vi "Gantry_GUI_Events.vi"(0 "COMPORT":refnum<visa-resource-name>="COM5", 5 "error in (no error)":errorcluster, 7 "Antenna Select":u16(ring)=1 items=["HOME", "TX1", "TX2", "TX3", "TX4", "TX5", "TX6", "TX7", "TX8", "TX9", "TX10", "TX11", "TX12", "RX8", "RX7", "RX6", "RX5", "RX4", "RX3", "RX2", "RX1"], 8 "EnableDriver(t)":bool=TRUE, 9 "z ref":dbl=21.0 format="%#_6f", 10 "Operation":u16(ring) items=["W/R", "RD ONLY", "WR ONLY"], 11 "Set-Z(Inches)":dbl=21.0 format="%#_6f") -> (14 "GantryGuiRefOut":refnum<vi>, 19 "error out":errorcluster)   [LabVIEW 2018]
uses:
  <vilib>/Utility/file.llb/Read Delimited Spreadsheet (DBL).vi
panel:
  in  "Exe_write":bool=TRUE
  in  "Exit":bool=TRUE
  out "Success?(t)":bool
  in  "Exe_ctrl":bool=TRUE
  in  "Set-zMach":dbl=21.0 format="%#_6f"
  out "Get-z":dbl=21.0 format="%#_6f"
  out "Get-y":dbl format="%#_13g"
  out "Get-x":dbl
  out "py path":path
  in  "Selector Control":T1(radio)
  out "comport":string
  in  "Close Serial(t)":bool
  in  "Set-y":dbl format="%#_13g"
  in  "Set-x":dbl
  in  "Coordinates Ref File":path=path "C:/RageATE/Instruments/Zaber Gantry/Labview Code from Colin/Gantry/antenna_cords-4.csv"
  out "begin":dbl=83230.42149349999 format="%_19f"
  out "List":dbl[][](array[numeric])=[[0.0, 0.0, 0.0, 247141.0, 0.0, 52711.0, 103619.0], [156330.0, 638961.0, 0.0, 247141.0, 0.0, 0.0, 103619.0], [193621.0, 638961.0, 0.0, 284432.0, 0.0, 0.0, 140910.0], [230912.0, 638961.0, 0.0, 321723.0, 0.0, 0.0, 178201.0], [268203.0, 638961.0, 0.0, 359014.0, 0.0, 0.0, 215492.0], [305494.0, 638961.0, 0.0, 396305.0, 0.0, 0.0, 252783.0], [342785.0, 638961.0, 0.0, 433596.0, 0.0, 0.0, 290074.0], [380076.0, 638961.0, 0.0, 470887.0, 0.0, 0.0, 327365.0], [417367.0, 638961.0, 0.0, 508178.0, 0.0, 0.0, 364656.0], [454658.0, 638961.0, 0.0, 545469.0, 0.0, 0.0, 401947.0], [491949.0, 638961.0, 0.0, 582760.0, 0.0, 0.0, 439238.0], [529240.0, 638961.0, 0.0, 620051.0, 0.0, 0.0, 476529.0], [566531.0, 638961.0, 0.0, 657342.0, 0.0, 0.0, 513820.0], [556452.0, 873796.0, 0.0, 647263.0, 0.0, 0.0, 503741.0], [500440.0, 873796.0, 0.0, 591251.0, 0.0, 0.0, 447729.0], [444428.0, 873796.0, 0.0, 535239.0, 0.0, 0.0, 391717.0], [388416.0, 873796.0, 0.0, 479227.0, 0.0, 0.0, 335705.0], [332404.0, 873796.0, 0.0, 423215.0, 0.0, 0.0, 279693.0], [276392.0, 873796.0, 0.0, 367203.0, 0.0, 0.0, 223681.0], [220380.0, 873796.0, 0.0, 311191.0, 0.0, 0.0, 167669.0], [164368.0, 873796.0, 0.0, 255179.0, 0.0, 0.0, 111657.0], [0.0, 0.0, 0.0, 0.0, 0.0, 0.0, 0.0], [0.0, 0.0, 0.0, 0.0, 0.0, 0.0, 0.0], [0.0, 0.0, 0.0, 0.0, 0.0, 0.0, 0.0]]
  # "X-Y Controls"
  # "Z Controls"
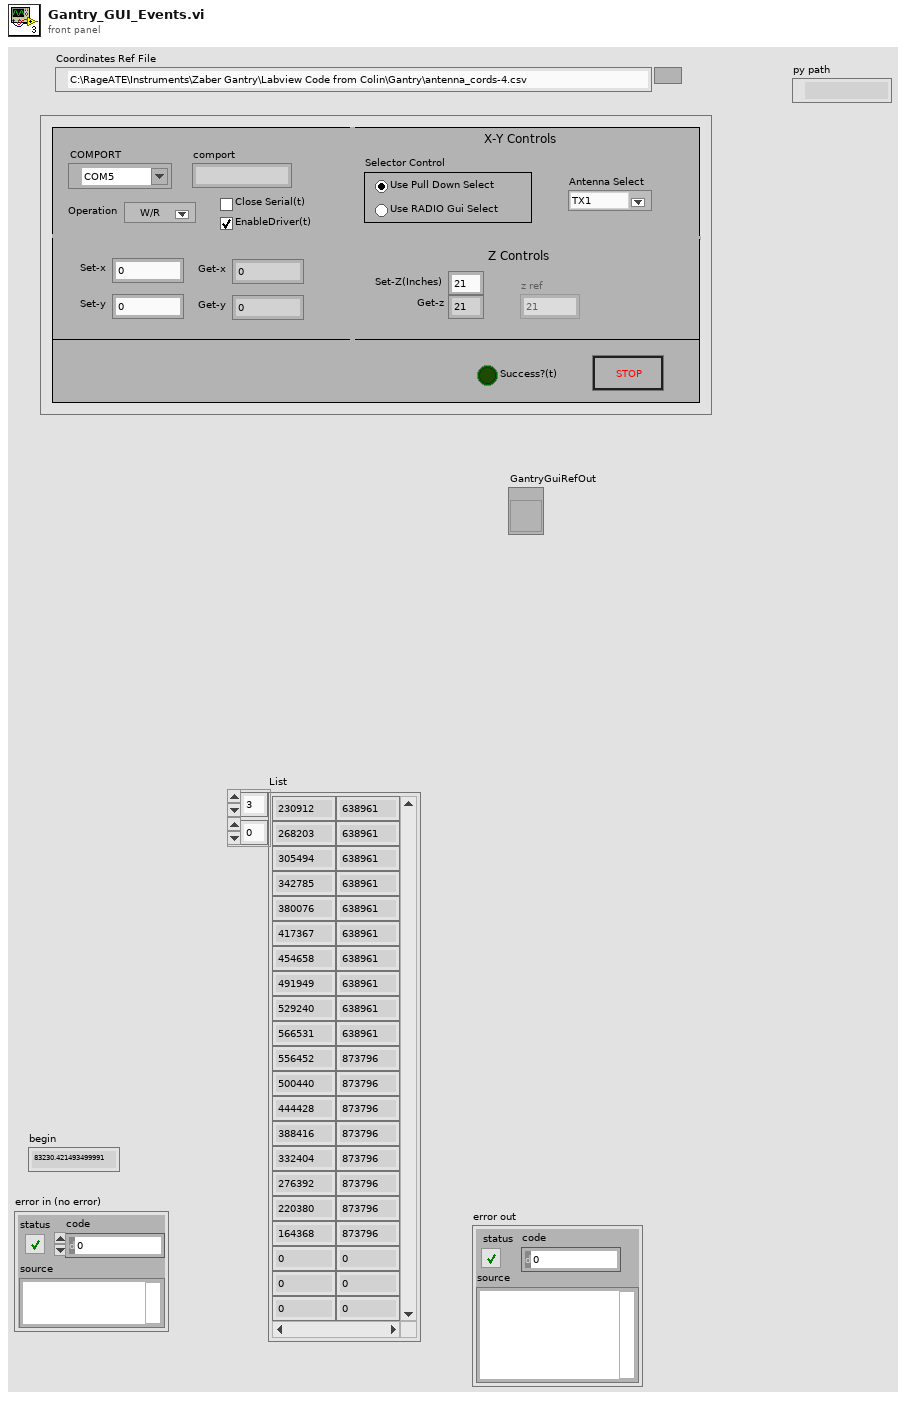
[diagram p1: front panel]
types:
  T1 = enum32{"Use Pull Down Select", "Use RADIO Gui Select"}
  T2 = enum8{"Enabled", "Disabled", "Disabled and Grayed Out"}
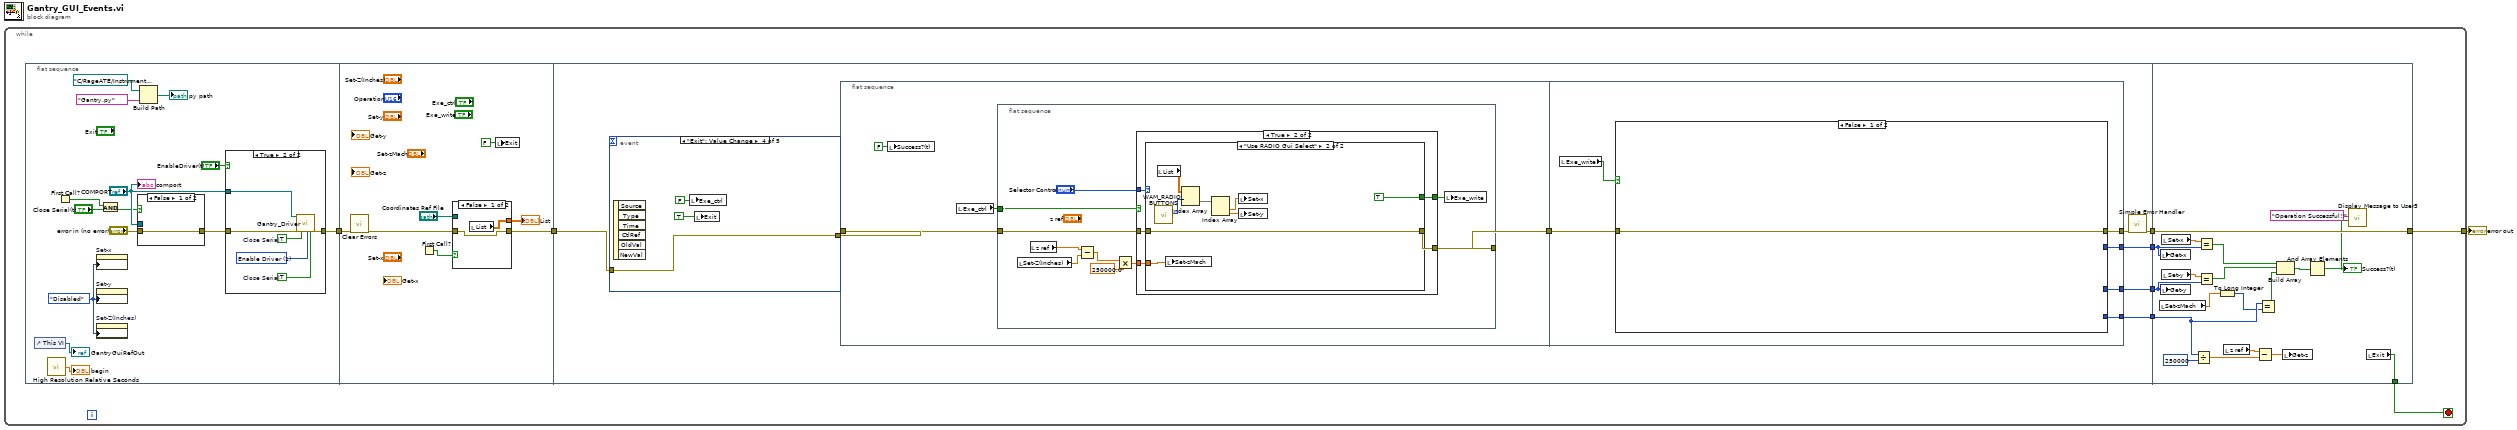
[diagram p0: block diagram]
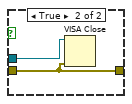
[diagram p2: hidden frame]
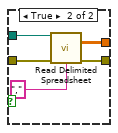
[diagram p4: hidden frame]
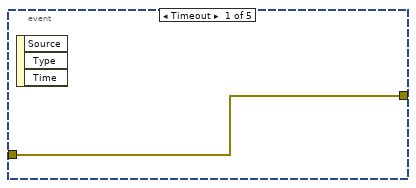
[diagram p5: hidden frame]
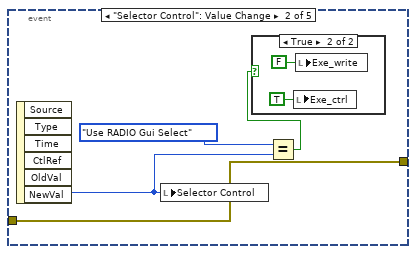
[diagram p6: hidden frame]
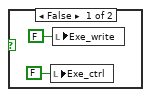
[diagram p7: hidden frame]
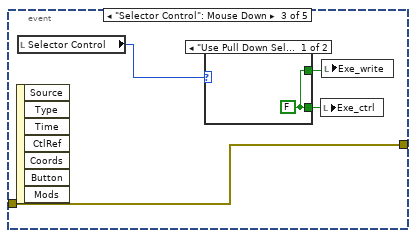
[diagram p8: hidden frame]
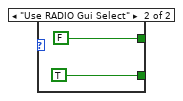
[diagram p9: hidden frame]
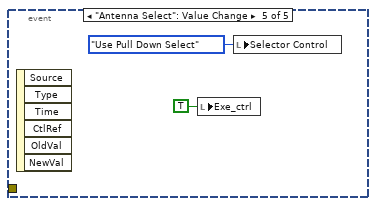
[diagram p10: hidden frame]
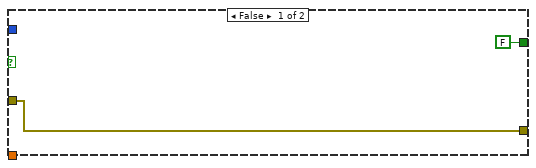
[diagram p11: hidden frame]
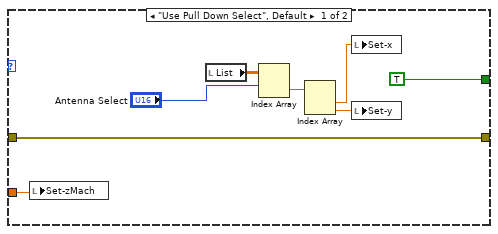
[diagram p12: hidden frame]
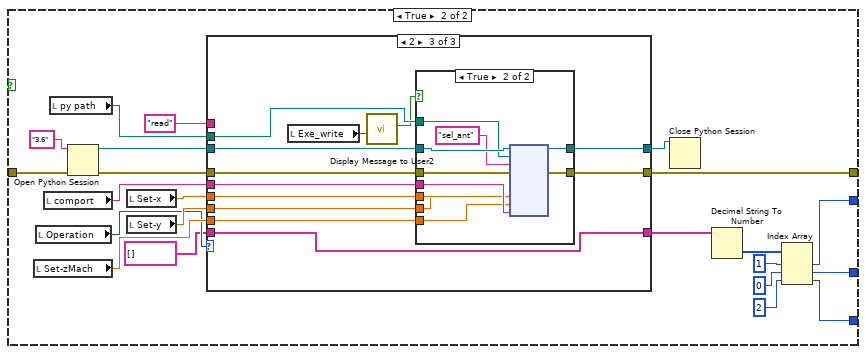
[diagram p13: hidden frame]
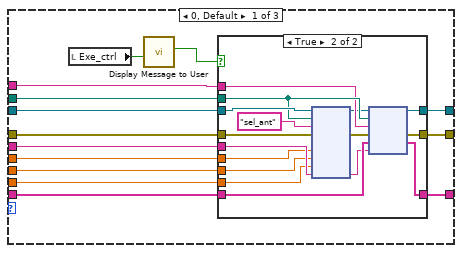
[diagram p14: hidden frame]
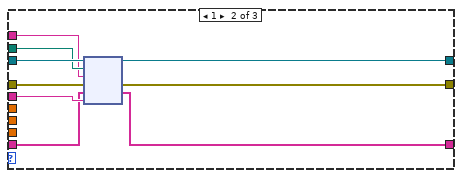
[diagram p16: hidden frame]
diagram:
  n1 = while {
    tunnel: [w3] -> w1
    stop <- w2 stop-if-true
    n2 = flat-sequence {
      tunnel: [w18] -> w9
      tunnel: w9 -> [w40]
      tunnel: [w36] -> w8
      tunnel: [w52] -> w7
      tunnel: [w55] -> w6
      tunnel: [w54] -> w5
      tunnel: [w51] -> w4
      tunnel: w8 -> [w48]
      tunnel: w7 -> [w227]
      tunnel: [w227] -> w3
      tunnel: w6 -> [w216]
      tunnel: w5 -> [w219]
      tunnel: w4 -> [w222]
      tunnel: [w211] -> w2
      frame #0 {
        w12 = T2."Disabled" ("Disabled")
        n3 = control-ref of="This VI"() -> (→"GantryGuiRefOut":refnum<vi>)
        n4 = call <vilib>:"High Resolution Relative Seconds.vi"() -> ("relative seconds"=→"begin":dbl)
        n5 = First Call?() -> (First Call?: T/F=w10:bool)
        n6 = property on="Set-x" class="DigNum (strict)"("DisabledEnum"=w12) -> ()  [unwired: 2 in, 2 out]
        n7 = property on="Set-y" class="DigNum (strict)"("DisabledEnum"=w12) -> ()  [unwired: 2 in, 2 out]
        n8 = property on="Set-Z(Inches)" class="DigNum (strict)"("DisabledEnum"=w12) -> ()  [unwired: 2 in, 2 out]
        n9 = And(x=w10, y="Close Serial(t)") -> (x .and. y?=w11:bool)
        n10 = case shown="False" w11 {
          tunnel: "error in (no error)" -> [w24 w25]
          tunnel: [w24 w25] -> w20
          tunnel: "COMPORT" -> [_ w26]
          frame False {
          }
          frame True {
            n11 = VISA Close(VISA resource name=w26, error in (no error)=w25) -> ()  [unwired: 1 out]
          }
        }
        n12 = Build Path(base path=path "C:/RageATE/Instruments/Zaber Gantry/Labview Code from Colin/Gantry" ("Driver Path"), name or relative path="Gantry.py") -> (appended path=→"py path":path)
        n13 = case shown="True" "EnableDriver(t)" {
          tunnel: "COMPORT" -> [_ w30]
          tunnel: w20 -> [w27 w33]
          tunnel: [w27 w29] -> w18
          frame False {
          }
          frame True {
            w28 = TRUE  # Close Serial
            w31 = u16 1 items=["Disable Driver", "Enable Driver", "Read Driver Status"] ("Driver-Func")
            w32 = TRUE  # Close Serial
            n14 = call "Gantry_Driver.vi"("VISA resource name"=w30, "error in (no error)"=w33, "Open Serial"=w32, "Driver-Func"=w31, "Close Serial"=w28) -> ("error out"=w29:errorcluster)  [unwired: 11 in, 3 out]
          }
        }
        "comport" <- "COMPORT"
      }
      frame #1 {
        n15 = call <vilib>:"Clear Errors.vi"("error in (no error)"=w40) -> ("error out"=w39:errorcluster)  [unwired: 5 in, 1 out]
        n16 = First Call?() -> (First Call?: T/F=w35:bool)
        n17 = case shown="False" w35 {
          tunnel: w39 -> [w41 w47]
          tunnel: "Coordinates Ref File" -> [_ w46]
          tunnel: [w42 w44] -> w37
          tunnel: [w41 w43] -> w36
          frame False {
            n18 = local read "List"() -> (w42:dbl[][])
          }
          frame True {
            n19 = call-poly <vilib>:"Read Delimited Spreadsheet.vi"("file path (dialog if empty)"=w46, "error in (no error)"=w47, "delimiter (\\t)"="," ("delimiter (\\t)")) -> ("all rows"=w44:dbl[][], "error out"=w43:errorcluster)  [unwired: 7 in, 4 out]
          }
        }
        "List" <- w37
        n20 = local write "Exit"(FALSE ("Exit")) -> ()
      }
      frame #2 {
        n21 = event shown="[3] \"Exit\": Value Change" {
          selector: _ -> [_ _ _ _ _]
          dyn-events: _ -> [_ _ _ _ _]
          timeout: _ -> [_ _ _ _ _]
          tunnel: w48 -> [w56 w60 w68 w72 _]
          tunnel: [w56 w60 w68 w72 _] -> w49
          event Timeout {
            n22 = event-data() -> ()  [unwired: 1 in, 3 out]
          }
          event "Selector Control": Value Change {
            n23 = event-data() -> ("NewVal"=w59:T1)  [unwired: 1 in, 5 out]
            n24 = local write "Selector Control"(w59) -> ()
            n25 = Equal?(x=T1."Use RADIO Gui Select", y=w59) -> (x = y?=w57:bool)
            n26 = case shown="True" w57 {
              frame False {
                n27 = local write "Exe_ctrl"(FALSE ("Exe_ctrl")) -> ()
                n28 = local write "Exe_write"(FALSE ("Exe_write")) -> ()
              }
              frame True {
                n29 = local write "Exe_ctrl"(TRUE ("Exe_ctrl")) -> ()
                n30 = local write "Exe_write"(FALSE ("Exe_write")) -> ()
              }
            }
          }
          event "Selector Control": Mouse Down {
            n31 = event-data() -> ()  [unwired: 1 in, 7 out]
            n32 = local read "Selector Control"() -> (w67:T1)
            n33 = case shown="\"Use Pull Down Select\", Default" w67 {
              tunnel: [w69 FALSE ("Exe_write")] -> w66
              tunnel: [w69 TRUE ("Exe_ctrl")] -> w65
              frame "Use Pull Down Select", Default {
                w69 = FALSE ("Exe_ctrl")
              }
              frame "Use RADIO Gui Select" {
              }
            }
            n34 = local write "Exe_ctrl"(w65) -> ()
            n35 = local write "Exe_write"(w66) -> ()
          }
          event "Exit": Value Change {
            n36 = event-data() -> ()  [unwired: 1 in, 6 out]
            n37 = local write "Exe_ctrl"(FALSE ("Execute")) -> ()
            n38 = local write "Exit"(TRUE ("Execute")) -> ()
          }
          event "Antenna Select": Value Change {
            n39 = event-data() -> ()  [unwired: 1 in, 6 out]
            n40 = local write "Exe_ctrl"(TRUE ("Execute")) -> ()
            n41 = local write "Selector Control"(T1."Use Pull Down Select" ("Selector Control")) -> ()
          }
        }
        n42 = flat-sequence {
          tunnel: w49 -> [w80]
          tunnel: [w79] -> w50
          tunnel: w50 -> [w119]
          tunnel: [w118] -> w54
          tunnel: [w117] -> w55
          tunnel: [w116] -> w51
          tunnel: [w115] -> w53
          frame #0 {
            n43 = local write "Success?(t)"(FALSE ("Success?(t)")) -> ()
            n44 = local read "Exe_ctrl"() -> (w78:bool)
            n45 = flat-sequence {
              tunnel: w80 -> [w90]
              tunnel: [w89] -> w79
              tunnel: w78 -> [w82]
              frame #0 {
                n46 = local read "Set-Z(Inches)"() -> (w86:dbl)
                n47 = local read "z ref"() -> (w88:dbl)
                n48 = Subtract(x=w88, y=w86) -> (x-y=w87:dbl)
                n49 = Multiply(x=w87, y=250000.0) -> (x*y=w84:dbl)
                n50 = case shown="True" w82 {
                  tunnel: w90 -> [w91 w97]
                  tunnel: [w91 w96] -> w89
                  tunnel: w84 -> [_ w95]
                  tunnel: [FALSE ("OK") w94] -> w83
                  tunnel: "Selector Control" -> [_ w93]
                  frame False {
                  }
                  frame True {
                    n51 = case shown="\"Use RADIO Gui Select\"" w93 {
                      tunnel: w97 -> [w98 w113]
                      tunnel: [w98 w113] -> w96
                      tunnel: w95 -> [w105 w107]
                      tunnel: [TRUE ("Execute") TRUE ("Execute")] -> w94
                      frame "Use Pull Down Select", Default {
                        n52 = local write "Set-zMach"(w105) -> ()
                        n53 = local read "List"() -> (w99:dbl[][])
                        n54 = Index Array(array=w99, index (row)="Antenna Select") -> (element=w101:dbl[])  [unwired: 1 in]
                        n55 = Index Array(array=w101) -> (element #1=w102:dbl, element #2=w103:dbl)  [unwired: 2 in]
                        n56 = local write "Set-x"(w102) -> ()
                        n57 = local write "Set-y"(w103) -> ()
                      }
                      frame "Use RADIO Gui Select" {
                        n58 = call "WAM_RADIO_BUTTONS.vi"() -> ("Index out"=w111:u32)  [unwired: 11 in]
                        n59 = local read "List"() -> (w112:dbl[][])
                        n60 = local write "Set-zMach"(w107) -> ()
                        n61 = Index Array(array=w112, index (row)=w111) -> (element=w110:dbl[])  [unwired: 1 in]
                        n62 = Index Array(array=w110) -> (element #1=w109:dbl, element #2=w108:dbl)  [unwired: 2 in]
                        n63 = local write "Set-x"(w109) -> ()
                        n64 = local write "Set-y"(w108) -> ()
                      }
                    }
                  }
                }
                n65 = local write "Exe_write"(w83) -> ()
              }
            }
          }
          frame #1 {
            n66 = local read "Exe_write"() -> (w114:bool)
            n67 = case shown="False" w114 {
              tunnel: w119 -> [w120 w138]
              tunnel: [_ w137] -> w118
              tunnel: [_ w136] -> w117
              tunnel: [_ w135] -> w116
              tunnel: [w120 w134] -> w115
              frame False {
              }
              frame True {
                n68 = local read "Set-zMach"() -> (w131:dbl)
                n69 = local read "Operation"() -> (w128:u16)
                n70 = local read "comport"() -> (w129:string)
                n71 = local read "py path"() -> (w130:path)
                n72 = Open Python Session(python version="3.6" ("Python version"), 3:w138) -> (session out=w125:refnum<k35>, error out=w126:errorcluster)  [unwired: 1 in]
                n73 = local read "Set-x"() -> (w132:dbl)
                n74 = local read "Set-y"() -> (w133:dbl)
                n75 = case shown="2" w128 {
                  tunnel: [w149 w182 w189] -> w124
                  tunnel: [w148 w183 w190] -> w134
                  tunnel: w130 -> [w154 w180 w194]
                  tunnel: w125 -> [w156 w181 w196]
                  tunnel: w126 -> [w155 w184 w195]
                  tunnel: w129 -> [w150 w179 w193]
                  tunnel: [w153 w178 w191] -> w127
                  tunnel: string[] [] -> [w152 w177 w191]
                  tunnel: "read" ("function name") -> [w151 w176 _]
                  tunnel: w131 -> [w147 _ w192]
                  tunnel: w132 -> [w146 _ w188]
                  tunnel: w133 -> [w145 _ w187]
                  frame 0, Default {
                    n76 = local read "Exe_ctrl"() -> (w143:bool)
                    n77 = call "Display Message to User"("Enable"=w143) -> ("OK"=w144:bool)  [unwired: 9 in, 1 out]
                    n78 = case shown="True" w144 {
                      tunnel: w156 -> [w158 w174]
                      tunnel: w155 -> [w159 w173]
                      tunnel: w154 -> [_ w172]
                      tunnel: [w157 w171] -> w153
                      tunnel: w152 -> [w157 w170]
                      tunnel: w151 -> [_ w169]
                      tunnel: w150 -> [_ w168]
                      tunnel: [w158 w166] -> w149
                      tunnel: [w159 w165] -> w148
                      tunnel: w147 -> [_ w164]
                      tunnel: w146 -> [_ w161]
                      tunnel: w145 -> [_ w160]
                      frame False {
                      }
                      frame True {
                        n79 = node(w174, w172, "sel_ant" ("function name"), w173, w161, w160, w164, w168) -> (w163:refnum<k35>, w162:errorcluster, w167:string)  [unwired: 5 in, 2 out]
                        n80 = node(w163, w172, w169, w162, w170, w167) -> (w166:refnum<k35>, w165:errorcluster, w171:string[])  [unwired: 1 in, 2 out]
                      }
                    }
                  }
                  frame 1 {
                    n81 = node(w181, w180, w176, w184, w177, w179) -> (w182:refnum<k35>, w183:errorcluster, w178:string[])  [unwired: 1 in, 2 out]
                  }
                  frame 2 {
                    n82 = local read "Exe_write"() -> (w185:bool)
                    n83 = call "Display Message to User2"("Enable"=w185) -> ("OK"=w186:bool)  [unwired: 9 in, 1 out]
                    n84 = case shown="True" w186 {
                      tunnel: w196 -> [w198 w208]
                      tunnel: w195 -> [w197 w207]
                      tunnel: w194 -> [_ w206]
                      tunnel: w193 -> [_ w205]
                      tunnel: w192 -> [_ w204]
                      tunnel: [w197 w203] -> w190
                      tunnel: [w198 w202] -> w189
                      tunnel: w188 -> [_ w201]
                      tunnel: w187 -> [_ w200]
                      frame False {
                      }
                      frame True {
                        n85 = node(w208, w206, "sel_ant" ("function name"), w207, w201, w200, w204, w205) -> (w202:refnum<k35>, w203:errorcluster)  [unwired: 6 in, 2 out]
                      }
                    }
                  }
                }
                n86 = Close Python Session(session in=w124) -> ()  [unwired: 1 in, 1 out]
                n87 = Decimal String To Number(string=w127) -> (number=w142:i32[])  [unwired: 2 in, 1 out]
                n88 = Index Array(array=w142, index #1=1 ("index"), index #2=0 ("index"), index #3=2 ("index")) -> (element #1=w137:i32, element #2=w136:i32, element #3=w135:i32)
              }
            }
          }
        }
        n89 = call <vilib>:"Simple Error Handler.vi"("error in (no error)"=w53) -> ("error out"=w52:errorcluster)  [unwired: 4 in, 4 out]
      }
      frame #3 {
        n90 = local read "Set-zMach"() -> (w221:dbl)
        n91 = local write "Get-x"(w219) -> ()
        n92 = local write "Get-y"(w216) -> ()
        n93 = local read "Set-x"() -> (w218:dbl)
        n94 = local read "Set-y"() -> (w217:dbl)
        n95 = Divide(x=w222, y=250000) -> (x/y=w223:dbl)
        n96 = Equal?(x=w218, y=w219) -> (x = y?=w214:bool)
        n97 = Equal?(x=w217, y=w216) -> (x = y?=w213:bool)
        n98 = To Long Integer(number=w221) -> (32bit integer=w220:i32)
        n99 = local read "z ref"() -> (w224:dbl)
        n100 = Subtract(x=w224, y=w223) -> (x-y=w226:dbl)
        n101 = Equal?(x=w222, y=w220) -> (x = y?=w212:bool)
        n102 = Build Array(w214, w213, w212) -> (w215:bool[])
        n103 = local write "Get-z"(w226) -> ()
        n104 = And Array Elements(Boolean array=w215) -> (logical AND=w210:bool)
        "Success?(t)" <- w210
        n105 = call "Display Message to User3"("Enable"=w210, "Message"="Operation Successful!!") -> ()  [unwired: 8 in, 2 out]
        n106 = local read "Exit"() -> (w211:bool)
      }
    }
  }
  "error out" <- w1
